vi "PV Heating-Cooling turbopump.vi"(8 "error in (no error)":errorcluster, 9 "PV Heating-Cooling - Cluster":T1={"Parameter"=0, "Parameter\nread only<->describe"=FALSE, "Pre-selection, heating\n  off     <-------->     on   "=TRUE, "TMS heating temperature\nset value [°C]"=40} {"TMS heating temperature\nset value [°C]" min=30 max=90 step=1; "Parameter" items=[" Pre-selection, heating [off / on]", " Heating TMS, actual value [°C] (read only)", " TMS regulator engaged [off/on] (read only)", " Maximum TMS temperature occured [°C] (read only)", " Heating type [conventional heating / TMS / cooling] (read only)", " TMS heating temperature set value [°C]"]}, 10 "Adress of unit":u16=1 min=1 max=999 step=1, 11 "VISA session":refnum<visa-resource-name>) -> (0 "error out":errorcluster, 2 "response (data)":string, 3 "dup VISA session":refnum<visa-resource-name>)   [LabVIEW 2021, in "Pfeiffer Vacuum.lvlib"]
doc: "There are 6 parameters available, only one of which can be enabled at a time. \n\n0 - Pre-selection, heating [off / on] (default) (Para.001)\n1 - Heating TMS, actual value [°C] (read only) (Para.331)\n2 - TMS regulator engaged [off/on] (read only) (Para.333)\n3 - Maximum TMS temperature occured [°C] (read only) (Para.334)\n4 - Heating type [conventional heating / TMS / cooling] (read only) (Para.335)\n5 - TMS heating temperature set value [°C] (Para.704)\n\nNote: The 2 controls right of this one will set the appropriate values for the selected parameter. Any settings for an parameter that is not selected will be ignored. If a value is out of range, it will be changed to either the upper or the lower limit of the range."
uses:
  <instrlib>/Pfeiffer Vacuum/Pfeiffer Vacuum.lvlib
  <instrlib>/Pfeiffer Vacuum/Public/Turbopumps/PV Heating-Cooling - Cluster.ctl
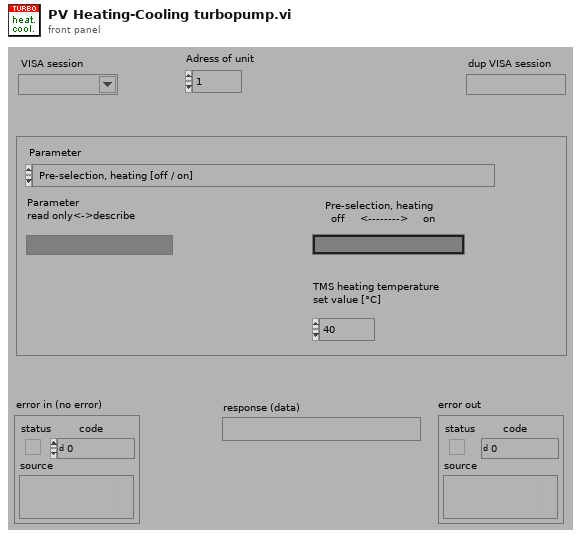
[diagram p1: front panel]
types:
  T1 = typedef "Pfeiffer Vacuum.lvlib/PV Heating-Cooling - Cluster.ctl" = cluster{"Parameter":u16, "Parameter\nread only<->describe":bool, "Pre-selection, heating\n  off     <-------->     on   ":bool, "TMS heating temperature\nset value [°C]":u16}
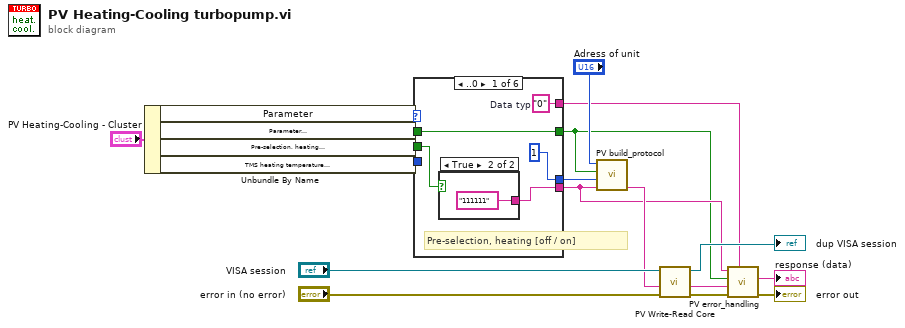
[diagram p0: block diagram]
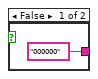
[diagram p2: hidden frame]
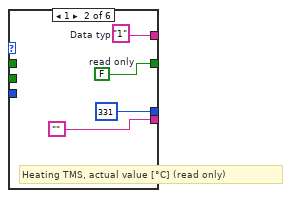
[diagram p3: hidden frame]
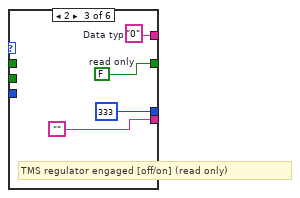
[diagram p4: hidden frame]
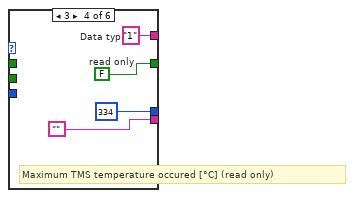
[diagram p5: hidden frame]
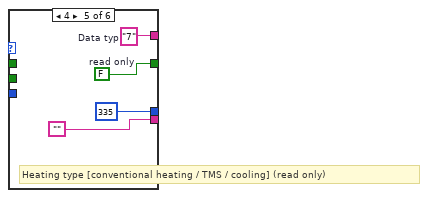
[diagram p6: hidden frame]
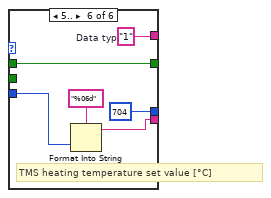
[diagram p7: hidden frame]
diagram:
  n1 = Unbundle By Name("PV Heating-Cooling - Cluster") -> ("Parameter"=w15:u16, "Parameter\nread only<->describe"=w14:bool, "Pre-selection, heating\n  off     <-------->     on"=w13:bool, "TMS heating temperature\nset value [°C]"=w12:u16)
  n2 = case shown="..0" w15 {
    tunnel: [u16 1 ("Parameter-number") u16 331 ("Parameter-number") u16 333 ("Parameter-number") u16 334 ("Parameter-number") u16 335 ("Parameter-number") u16 704 ("Parameter-number")] -> w17
    tunnel: [w22 "" "" "" "" w45] -> w2
    tunnel: [w21 w28 w32 w36 w40 w46] -> w1
    tunnel: w14 -> [w21 _ _ _ _ w46]
    tunnel: w13 -> [w20 _ _ _ _ _]
    tunnel: w12 -> [_ _ _ _ _ w44]
    tunnel: [w19 w26 w30 w34 w38 w42] -> w3
    frame ..0 {
      w19 = "0"  # Data typ
      # "Pre-selection, heating [off / on]"
      n3 = case shown="True" w20 {
        tunnel: ["000000" ("Data") "111111" ("Data")] -> w22
        frame False {
        }
        frame True {
        }
      }
    }
    frame 1 {
      w26 = "1"  # Data typ
      w28 = FALSE  # read only
      # "Heating TMS, actual value [°C] (read only)"
    }
    frame 2 {
      w30 = "0"  # Data typ
      w32 = FALSE  # read only
      # "TMS regulator engaged [off/on] (read only)"
    }
    frame 3 {
      w34 = "1"  # Data typ
      w36 = FALSE  # read only
      # "Maximum TMS temperature occured [°C] (read only)"
    }
    frame 4 {
      w38 = "7"  # Data typ
      w40 = FALSE  # read only
      # "Heating type [conventional heating / TMS / cooling] (read only)"
    }
    frame 5.. {
      w42 = "1"  # Data typ
      # "TMS heating temperature set value [°C]"
      n4 = Format Into String(format string="%06d" ("Format-String"), w44) -> (resulting string=w45:string)  [unwired: 2 in, 1 out]
    }
  }
  n5 = call <instrlib>:"PV build_protocol.vi"("Data"=w2, "Parameter-number"=w17, "parameter\nread<->describe"=w1, "Adress"="Adress of unit") -> ("output"=w9:string)  [unwired: 3 in]
  n6 = call <instrlib>:"PV Write-Read Core.vi"("error in"="error in (no error)", "Write data in"=w9, "VISA session"="VISA session") -> ("error out"=w7:errorcluster, "response (data) out"=w8:string, "dup VISA session"=→"dup VISA session":refnum<visa-resource-name>)  [unwired: 2 in]
  n7 = call <instrlib>:"PV error_handling.vi"("Data Typ in"=w3, "error in"=w7, "response (data) in"=w8, "Parameter\nread only<->describe"=w1, "data in"=w2) -> ("error out"=→"error out":errorcluster, "Data out"=→"response (data)":string)  [unwired: 4 in, 1 out]
